vi "Teleop.vi"(10 "Match Info":T1={"Autonomous Elapsed Seconds"=0.0, "TeleOp Elapsed Seconds"=0.0, "Disabled Elapsed Seconds"=0.0, "Visited Autonomous"=FALSE, "Visited TeleOp"=FALSE, "Visited Disabled"=FALSE, "Autonomous Settings"={"Autonomous Style"=enum."Independent", "VI Refnum"=refnum}}, 11 "Call Context":T2) -> ()   [LabVIEW 2015]
doc: "This VI is called for each TeleOp packet received from the DS where the robot is not disabled. It is often used to read from the joysticks and update I/O or to update setpoints for timed control loops. It should complete and return within 20 milliseconds or it may miss DS packets."
uses:
  <vilib>/Rock Robotics/WPI/DriverStation/WPI_DriverStationDerivedRobotMode.ctl
  <vilib>/Rock Robotics/WPI/DriverStation/WPI_DriverStationMatch Info.ctl
  <vilib>/Rock Robotics/WPI/Utilities/WPI_GetSetVariantRefNum.vi
  Robot Global Data.vi
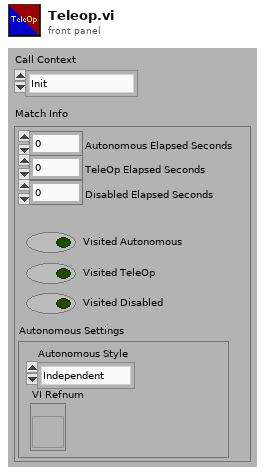
[diagram p1: front panel]
types:
  T1 = typedef "WPI_DriverStationMatch Info.ctl" = cluster{"Autonomous Elapsed Seconds":dbl, "TeleOp Elapsed Seconds":dbl, "Disabled Elapsed Seconds":dbl, "Visited Autonomous":bool, "Visited TeleOp":bool, "Visited Disabled":bool, "Autonomous Settings":cluster{"Autonomous Style":enum16{"Iterative", "Independent"}, "VI Refnum":refnum<vi>}}
  T2 = typedef "WPI_DriverStationDerivedRobotMode.ctl" = enum16{"Init", "Execute", "Stop"}
  T3 = typedef "WPI_JoystickDevRef.ctl" = cluster{"Device":T4}
  T4 = typedef "WPI_JoystickDeviceEnum.ctl" = enum16{"USB 0", "USB 1", "USB 2", "USB 3", "USB 4", "USB 5"}
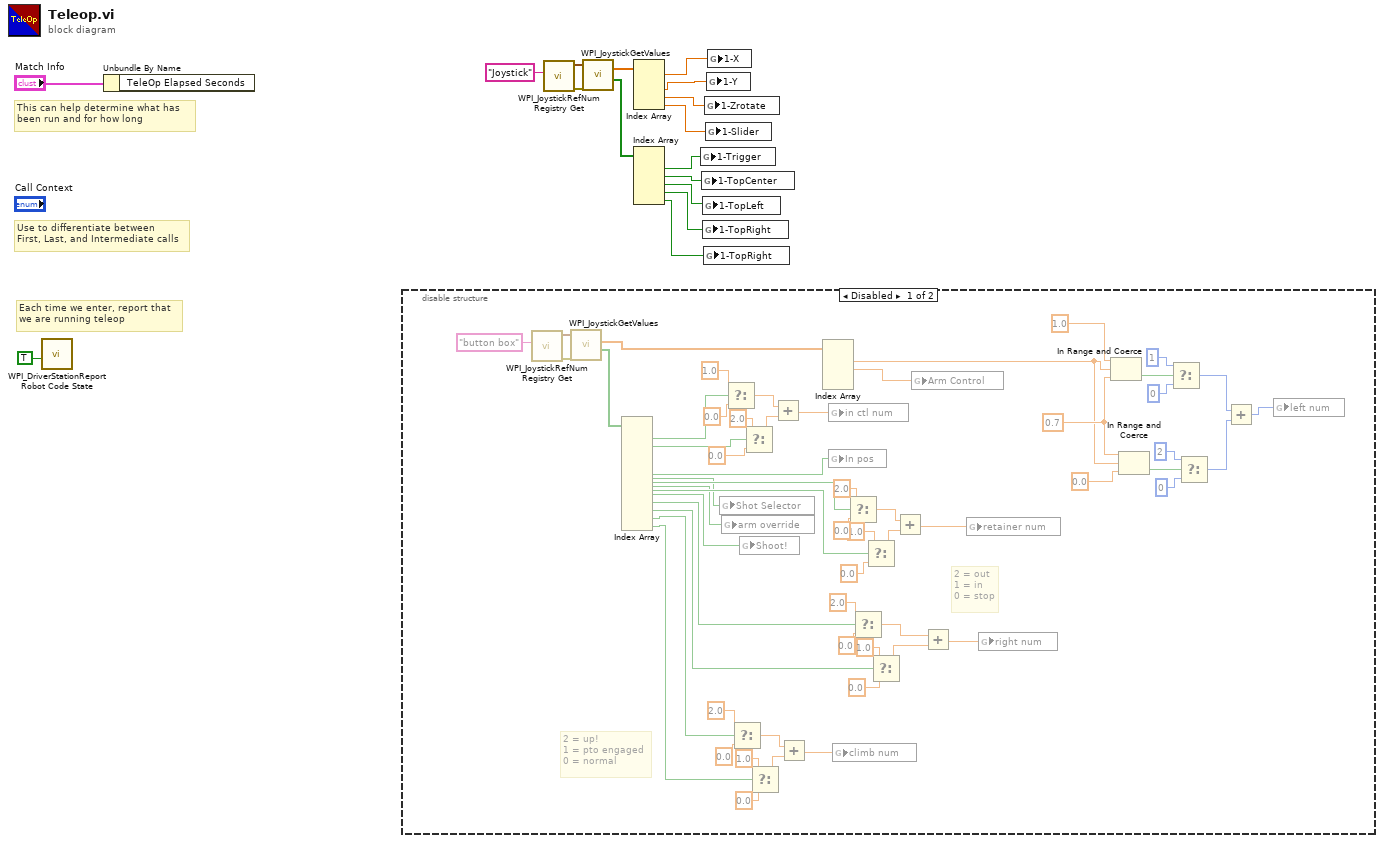
[diagram p0: block diagram]
diagram:
  # "Each time we enter, report that\nwe are running teleop"
  # "Use to differentiate between\nFirst, Last, and Intermediate calls"
  # "This can help determine what has\nbeen run and for how long"
  n1 = call <vilib>:"WPI_DriverStationReport Robot Code State.vi"("TeleOp"=TRUE ("Autonomous")) -> ()  [unwired: 10 in, 1 out]
  n2 = Unbundle By Name("Match Info") -> ()  [unwired: 1 out]
  n3 = disable-structure shown="Disabled" {
    frame Disabled {
      w31 = 0.7 ("upper limit")
      # "2 = up!\n1 = pto engaged\n0 = normal"
      # "2 = out\n1 = in\n0 = stop"
      n4 = call <vilib>:"WPI_JoystickRefNum Registry Get.vi"("refnum name"="button box") -> ("error out"=w74:errorcluster, "JoystickDevRef"=w73:T3)  [unwired: 9 in]
      n5 = call <vilib>:"WPI_JoystickGetValues.vi"("error in (no error)"=w74, "JoystickDevRef"=w73) -> ("Buttons"=w72:bool[], "Axes"=w46:dbl[])  [unwired: 5 in, 3 out]
      n6 = Index Array(array=w72) -> (element #1=w65:bool, element #2=w64:bool, element #3=w63:bool, element #4=w58:bool, element #5=w57:bool, element #6=w56:bool, element #7=w55:bool, element #8=w54:bool, element #9=w48:bool, element #10=w47:bool, element #11=w40:bool, element #12=w39:bool)  [unwired: 12 in]
      n7 = global write "Robot Global Data.vi" "Shot Selector"(w56) -> ()
      n8 = global write "Robot Global Data.vi" "arm override"(w55) -> ()
      n9 = Select(t=1.0, s=w65, f=0.0) -> (s? t:f=w67:dbl)
      n10 = Select(t=2.0, s=w40, f=0.0) -> (s? t:f=w42:dbl)
      n11 = global write "Robot Global Data.vi" "Shoot!"(w54) -> ()
      n12 = Select(t=2.0, s=w64, f=0.0) -> (s? t:f=w68:dbl)
      n13 = Select(t=1.0, s=w39, f=0.0) -> (s? t:f=w43:dbl)
      n14 = Add(x=w67, y=w68) -> (x+y=w66:dbl)
      n15 = Add(x=w42, y=w43) -> (x+y=w41:dbl)
      n16 = Index Array(array=w46) -> (element #1=w28:dbl, element #2=w38:dbl)  [unwired: 4 in, 2 out]
      n17 = global write "Robot Global Data.vi" "in ctl num"(w66) -> ()
      n18 = global write "Robot Global Data.vi" "In pos"(w63) -> ()
      n19 = global write "Robot Global Data.vi" "climb num"(w41) -> ()
      n20 = Select(t=2.0, s=w58, f=0.0) -> (s? t:f=w60:dbl)
      n21 = Select(t=2.0, s=w48, f=0.0) -> (s? t:f=w50:dbl)
      n22 = Select(t=1.0, s=w57, f=0.0) -> (s? t:f=w61:dbl)
      n23 = Select(t=1.0, s=w47, f=0.0) -> (s? t:f=w51:dbl)
      n24 = Add(x=w60, y=w61) -> (x+y=w59:dbl)
      n25 = global write "Robot Global Data.vi" "Arm Control"(w38) -> ()
      n26 = Add(x=w50, y=w51) -> (x+y=w49:dbl)
      n27 = global write "Robot Global Data.vi" "retainer num"(w59) -> ()
      n28 = global write "Robot Global Data.vi" "right num"(w49) -> ()
      n29 = In Range and Coerce(upper limit=1.0, x=w28, lower limit=w31) -> (In Range?=w34:bool)  [unwired: 1 out]
      n30 = In Range and Coerce(upper limit=w31, x=w28, lower limit=0.0) -> (In Range?=w37:bool)  [unwired: 1 out]
      n31 = Select(t=i8 1, s=w34, f=i8 0) -> (s? t:f=w26:i8)
      n32 = Select(t=i8 2, s=w37, f=i8 0) -> (s? t:f=w25:i8)
      n33 = Add(x=w26, y=w25) -> (x+y=w27:i8)
      n34 = global write "Robot Global Data.vi" "left num"(w27) -> ()
    }
    frame Enabled {
    }
  }
  n35 = call <vilib>:"WPI_JoystickRefNum Registry Get.vi"("refnum name"="Joystick") -> ("error out"=w13:errorcluster, "JoystickDevRef"=w12:T3)  [unwired: 9 in]
  n36 = call <vilib>:"WPI_JoystickGetValues.vi"("error in (no error)"=w13, "JoystickDevRef"=w12) -> ("Buttons"=w9:bool[], "Axes"=w11:dbl[])  [unwired: 5 in, 3 out]
  n37 = Index Array(array=w11) -> (element #1=w1:dbl, element #2=w2:dbl, element #3=w10:dbl, element #4=w6:dbl)  [unwired: 4 in]
  n38 = Index Array(array=w9) -> (element #1=w8:bool, element #2=w4:bool, element #3=w7:bool, element #4=w5:bool, element #5=w3:bool)  [unwired: 5 in]
  n39 = global write "Robot Global Data.vi" "1-Trigger"(w8) -> ()
  n40 = global write "Robot Global Data.vi" "1-TopCenter"(w4) -> ()
  n41 = global write "Robot Global Data.vi" "1-TopLeft"(w7) -> ()
  n42 = global write "Robot Global Data.vi" "1-TopRight"(w5) -> ()
  n43 = global write "Robot Global Data.vi" "1-TopRight"(w3) -> ()
  n44 = global write "Robot Global Data.vi" "1-Zrotate"(w10) -> ()
  n45 = global write "Robot Global Data.vi" "1-Slider"(w6) -> ()
  n46 = global write "Robot Global Data.vi" "1-Y"(w2) -> ()
  n47 = global write "Robot Global Data.vi" "1-X"(w1) -> ()
